vi "OMV_Simpletest.vi"() -> ()   [LabVIEW 2020]
panel:
  out "String":string
  in  "stop":bool
  out "Errors":string
  out "Version":string
  in  "VISA resource name":refnum<visa-resource-name>="ASRL30::INSTR"
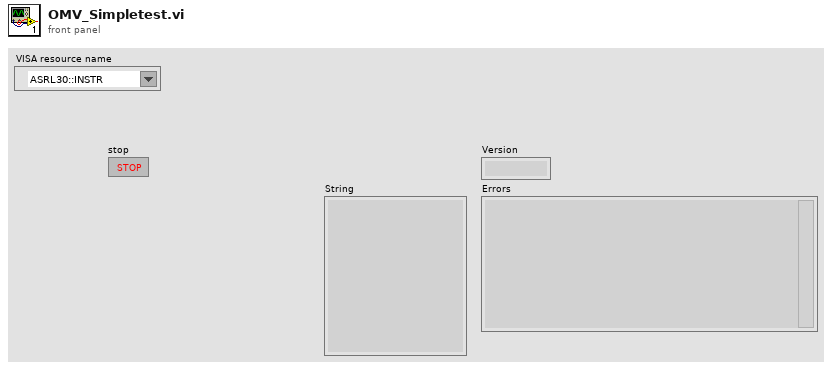
[diagram p1: front panel]
types:
  T1 = typedef "PythonCtrl.ctl" = cluster{"session":refnum<k35>, "PyPath":path, "Processor":T2}
  T2 = typedef "Processors.ctl" = enum16{"SPIKE", "Pi", "Pi_ssh", "OpenMV"}
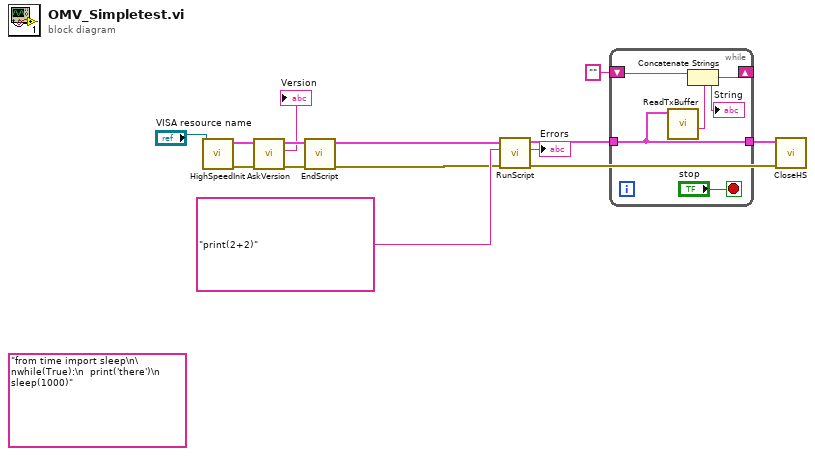
[diagram p0: block diagram]
diagram:
  (unwired) "from time import sleep\n\nwhile(True):\n  print('there')\n  sleep(1000)" ("header buffer")
  n1 = call "HighSpeedInit.vi"("Python"="VISA resource name") -> ("error out"=w13:errorcluster, "Python"=w12:T1)  [unwired: 9 in]
  n2 = call "AskVersion.vi"("error in"=w13, "Python"=w12) -> ("error out"=w11:errorcluster, "Version"=→"Version":string, "Python"=w10:T1)  [unwired: 7 in]
  n3 = call "EndScript.vi"("error in (no error)"=w11, "Python"=w10) -> ("error out"=w8:errorcluster, "Python"=w1:T1)  [unwired: 7 in, 1 out]
  n4 = call "RunScript.vi"("error in"=w8, "script"="print(2+2)" ("header buffer"), "Python"=w1) -> ("error out"=w6:errorcluster, "Tx"=→"Errors":string, "Python"=w3:T1)  [unwired: 6 in]
  n5 = while {
    tunnel: [w18] -> w4
    tunnel: w3 -> [w18]
    shift-right: [w15] -> _
    shift-left: "" -> [w17]
    stop <- "stop" stop-if-true
    n6 = call "ReadTxBuffer.vi"("Python"=w18) -> ("Tx Buffer"=w16:string)  [unwired: 7 in, 3 out]
    n7 = Concatenate Strings(w17, w16) -> (w15:string)
    "String" <- w15
  }
  n8 = call "CloseHS.vi"("error in (no error)"=w6, "Python"=w4) -> ()  [unwired: 10 in]
